vi "Access Platform DB Path.vi"(11 "名称或相对路径":string="database1.mdb") -> (2 "Connection information":string, 3 "Path out":string)   [LabVIEW 2016, in "Access Lib.lvlib"]
uses:
  Access Lib.lvlib
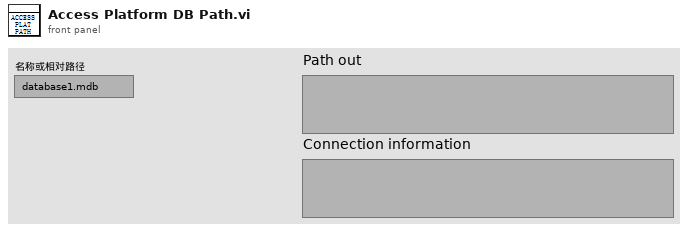
[diagram p1: front panel]
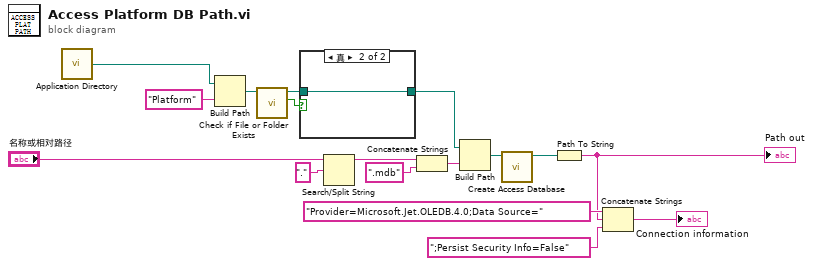
[diagram p0: block diagram]
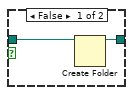
[diagram p2: hidden frame]
diagram:
  n1 = call <vilib>:"Application Directory.vi"() -> ("Application Directory"=w1:path)
  n2 = Build Path(base path=w1, name or relative path="Platform" ("名称或相对路径")) -> (appended path=w13:path)
  n3 = call <vilib>:"Check if File or Folder Exists.vi"("path"=w13) -> ("file or folder exists?"=w17:bool, "dup path"=w16:path)  [unwired: 8 in, 1 out]
  n4 = case shown="真" w17 {
    tunnel: w16 -> [w19 w20]
    tunnel: [w18 w20] -> w15
    frame False {
      n5 = Create Folder(path (use dialog)=w19) -> (created path=w18:path)  [unwired: 2 in, 2 out]
    }
    frame True {
    }
  }
  n6 = Search/Split String(string="名称或相对路径", search string/char (-)="." ("搜索字符串/字符(-)")) -> (substring before match=w11:string)  [unwired: 1 in, 2 out]
  n7 = Concatenate Strings(w11, ".mdb" ("字符串")) -> (w7:string)
  n8 = Build Path(base path=w15, name or relative path=w7) -> (appended path=w12:path)
  n9 = call "Create Access Database.vi"("路径"=w12) -> ("路径 out"=w4:path)  [unwired: 9 in, 1 out]
  n10 = Path To String(path=w4) -> (string=w3:string)
  "Path out" <- w3
  n11 = Concatenate Strings("Provider=Microsoft.Jet.OLEDB.4.0;Data Source=" ("condition"), w3, ";Persist Security Info=False" ("condition")) -> (→"Connection information":string)
